vi "Main.vi"(0 "Page Selector":T1, 1 "Code":i32 min=0 max=40000, 5 "Mode Selector":T3, 7 "Instrument Setting":T4={"Error Percentage"=20.0}, 9 "INL Method":T5, 11 "Error In":errorcluster, 12 "Input Voltage Parameters":T6={"Voltage Max"=5.0, "Voltage Min"=0.0, "Resolution (Bits)"=3}) -> (3 "DNL Value":dbl, 4 "Tab Control":T2(tab), 6 "DNL Graph":dbl[](graph), 8 "INL Graph":dbl[](graph), 10 "Ideal Transfer Function":cluster{"Analog Voltage":dbl[], dbl[]}(graph), 13 "INL Value":dbl, 14 "Status":string, 15 "Error Out":errorcluster)   [LabVIEW 2023]
uses:
  Typedef/INL Method.ctl
  Typedef/Page Selector.ctl
  Typedef/Mode Selector.ctl
  Typedef/Input Values.ctl
  Typedef/Instrument Setting.ctl
  Typedef/Queue Operation.ctl
  Typedef/INL DNL Data.ctl
  Classes/Application/Application.lvclass
  Typedef/DVR ref.ctl
  Typedef/User Event Operations.ctl
panel:
  in  "Input":bool
  # "INL AND DNL TESTING INSTRUMENT"
  # "Purpose\nThis tool measures Integral Non-Linearity (INL) and Differential Non-Linearity (DNL) of ADCs and DACs, ensuring accurate linearity performance for various applications.\n\nINL and DNL Definitions\nINL (Integral Non-Linearity): Deviation of the converter's actual transfer function from an ideal straight line.\nDNL (Differential Non-Linearity): Deviation between adjacent digital output levels, indicating the uniformity of steps.\n\nHow to Use\nMode Selection: Choose DAC or ADC.\nInput Parameters: Enter voltage range and bit resolution.\nConfigure Settings: Set error percentage and INL measurement method.\nRun Measurements: View DNL and INL results in real-time."
  # "Please select the mode of the device"
  # "Choose the type of INL Measurement"
  # "Please enter the input voltage parameters to generate ideal transfer function"
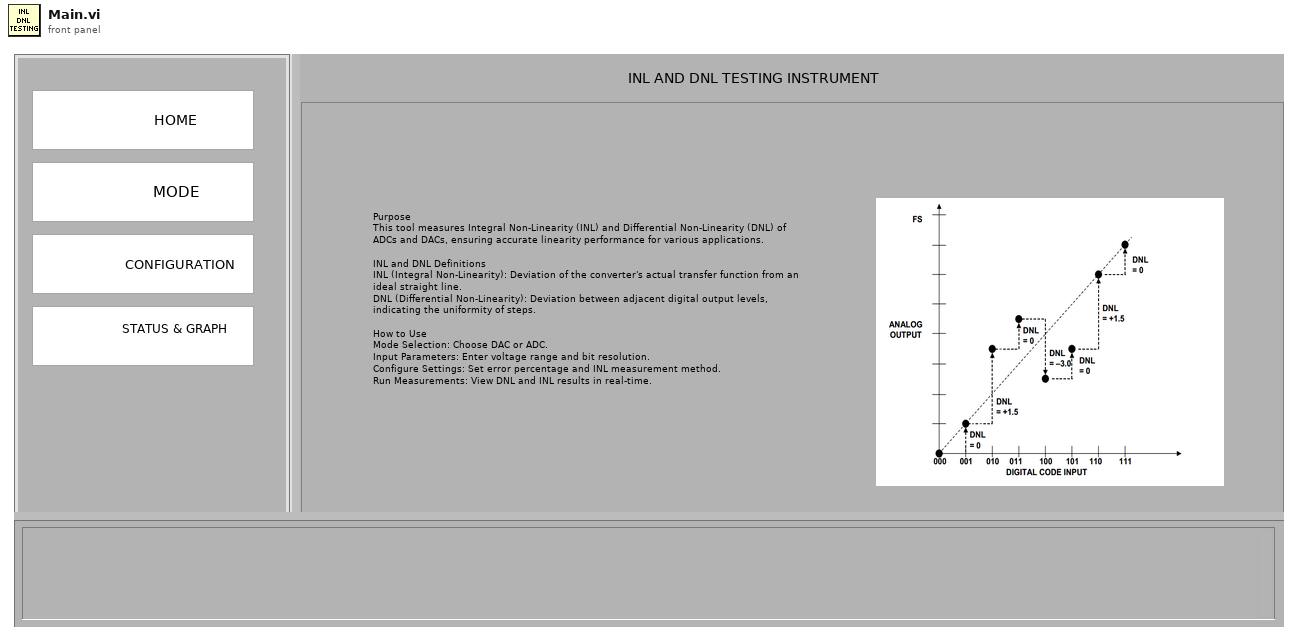
[diagram p1: front panel]
types:
  T1 = typedef "Page Selector.ctl" = cluster{"Mode":bool, "Configuration":bool, "Result":bool, "Home":bool}
  T2 = enum32{"Home Page", "Mode Page", "Configuration Page", "Input Page", "Result Page"}
  T3 = typedef "Mode Selector.ctl" = cluster{"DAC":bool, "ADC":bool}
  T4 = typedef "Instrument Setting.ctl" = cluster{"Error Percentage":dbl}
  T5 = typedef "INL Method.ctl" = enum16{"Best Fit", "End Point"}
  T6 = typedef "Input Values.ctl" = cluster{"Voltage Max":dbl, "Voltage Min":dbl, "Resolution (Bits)":i32}
  T7 = typedef "User Event Operations.ctl" = enum16{"Obtain", "Generate", "Destroy"}
  T8 = typedef "INL DNL Data.ctl" = cluster{"Page":enum32{"Home Page", "Mode Page", "Configuration Page", "Input Page", "Result Page"}, "Voltage Range":dbl, "Input Values":T6, "LSB":dbl, "Analog Voltage":dbl[], "Digital Code":dbl[], "TF Graph":cluster{"Analog Voltage":dbl[], dbl[]}, "DNL":dbl, "INL":dbl, "DNL Graph":dbl[], "Code":i32, "Actual Voltage":dbl[], "INL Graph":dbl[], "V Zero":dbl, "Error Percentage":dbl, "Status Array":string[], "Status Limit":i32, "Statusbar":string, "Active Class":refnum<class "Application.lvclass">, "INL Method":T5, "List of Classes":T9[], "Selected Mode":string, "Base Class":refnum<class "Application.lvclass">}
  T9 = typedef "DVR ref.ctl" = cluster{"Class Name":string, "Class Data":refnum<class "Application.lvclass">}
  T10 = typedef "Queue Operation.ctl" = enum16{"Create & Enqueue N", "Enqueue N", "Dequeue", "Enstack N", "Flush", "Release"}
  T11 = typedef "Queue Element.ctl" = cluster{"State":string, "Data":variant}
  T12 = typedef "Transfer Function.ctl" = cluster{"Ideal voltage":dbl[], "Digital Code":dbl[]}
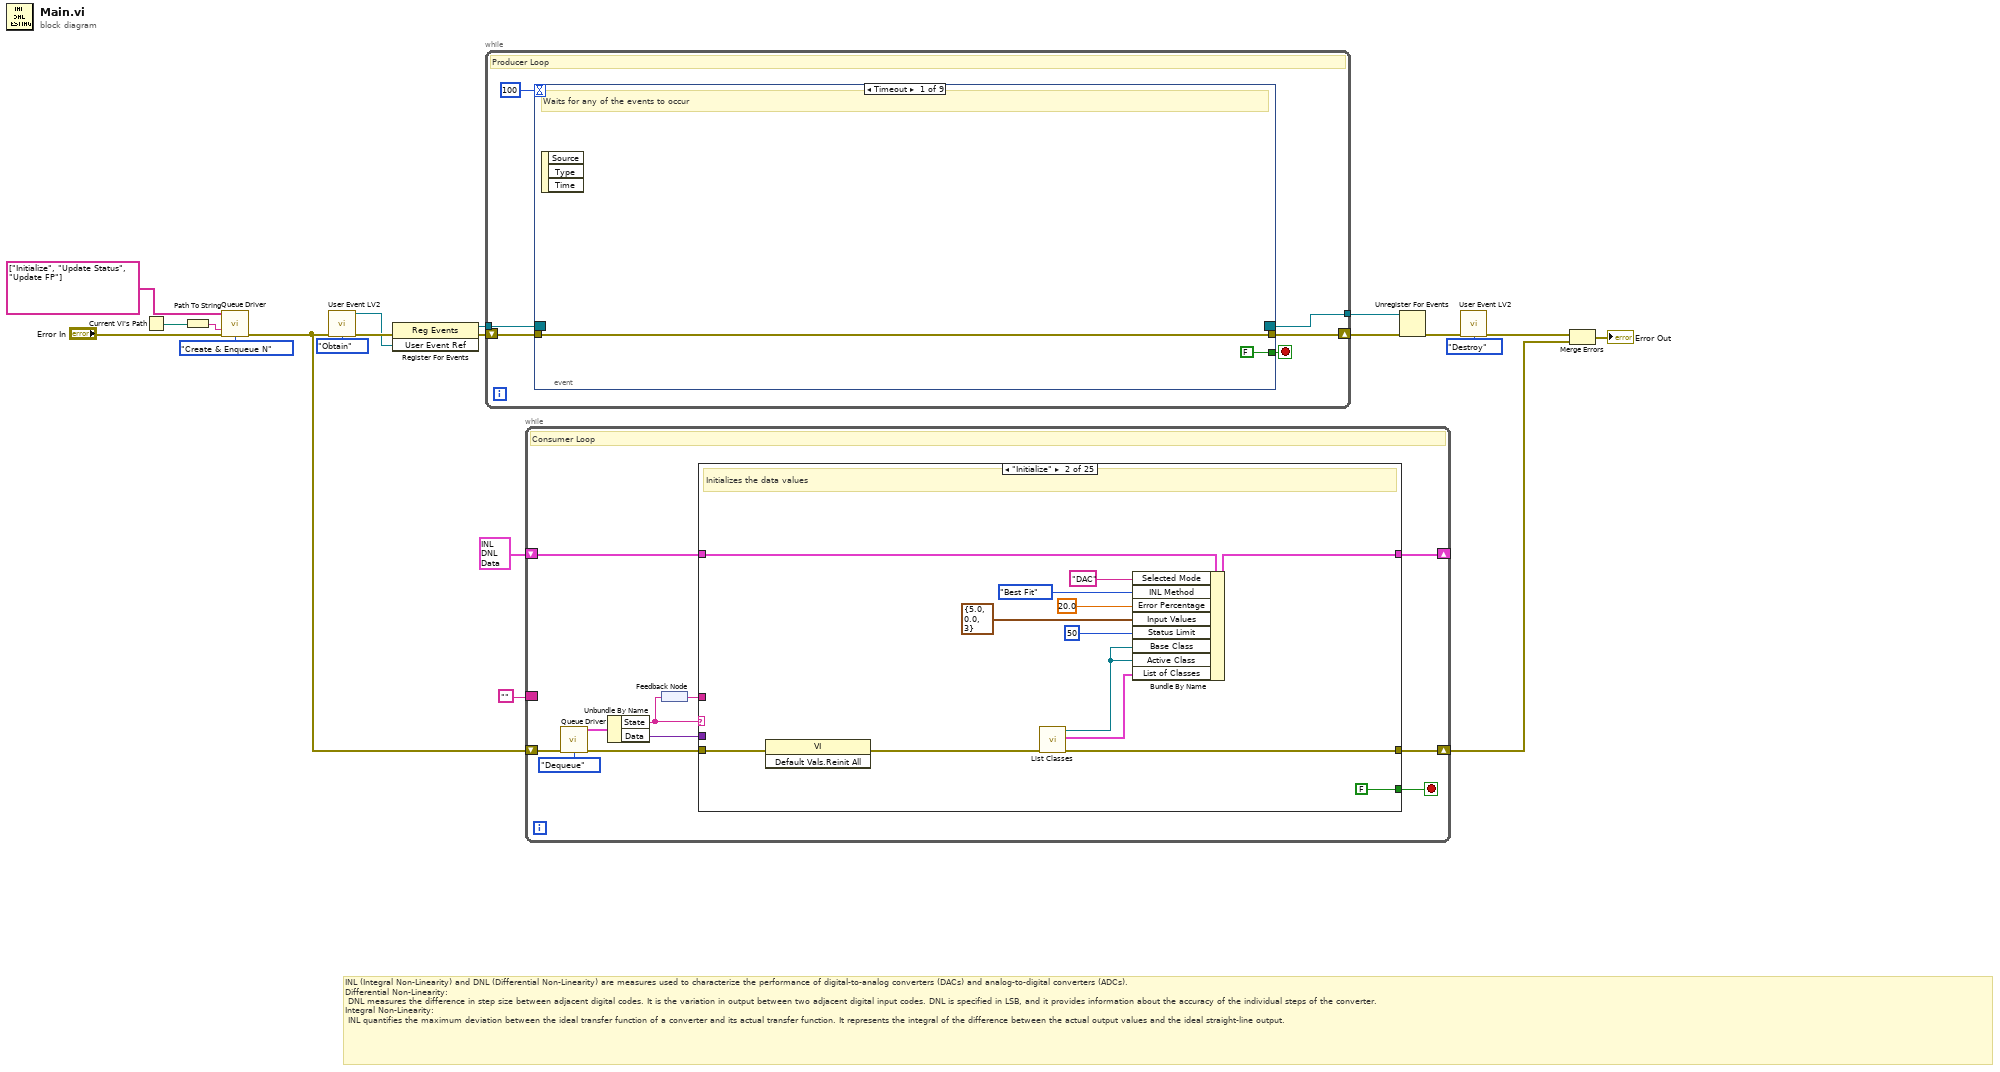
[diagram p0: block diagram]
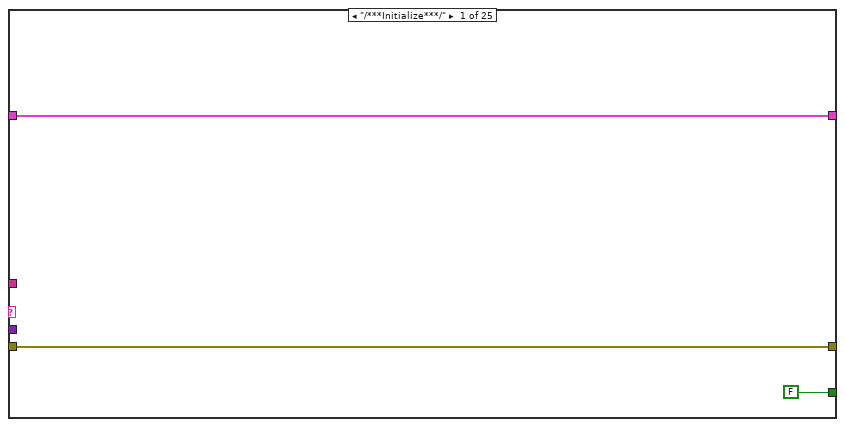
[diagram p2: hidden frame]
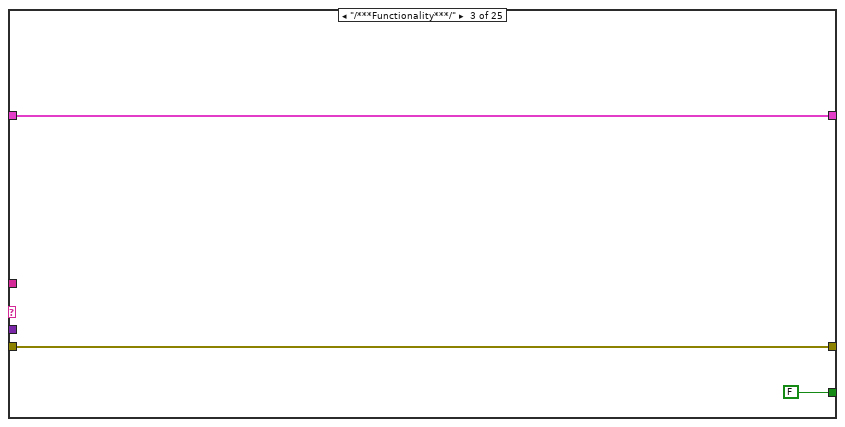
[diagram p3: hidden frame]
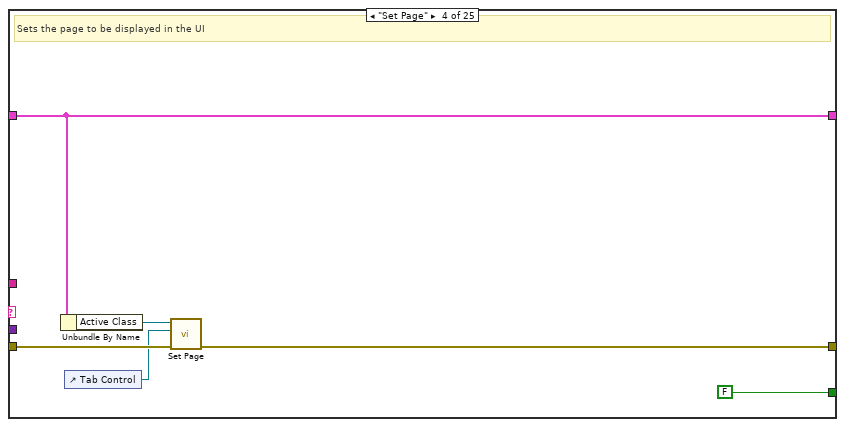
[diagram p4: hidden frame]
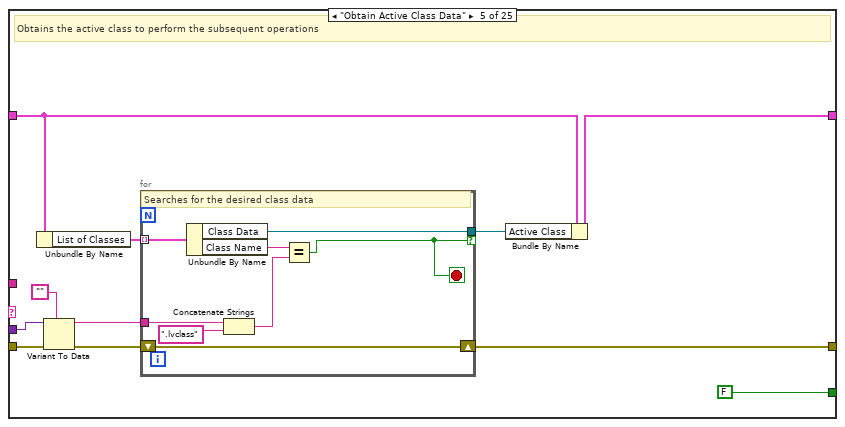
[diagram p5: hidden frame]
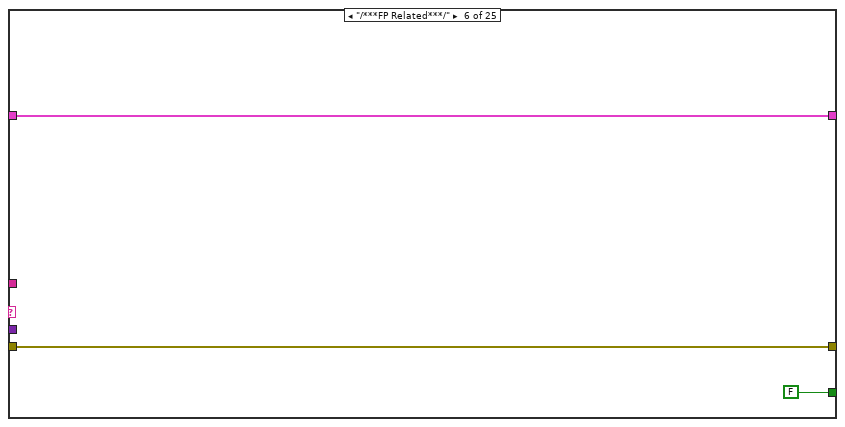
[diagram p6: hidden frame]
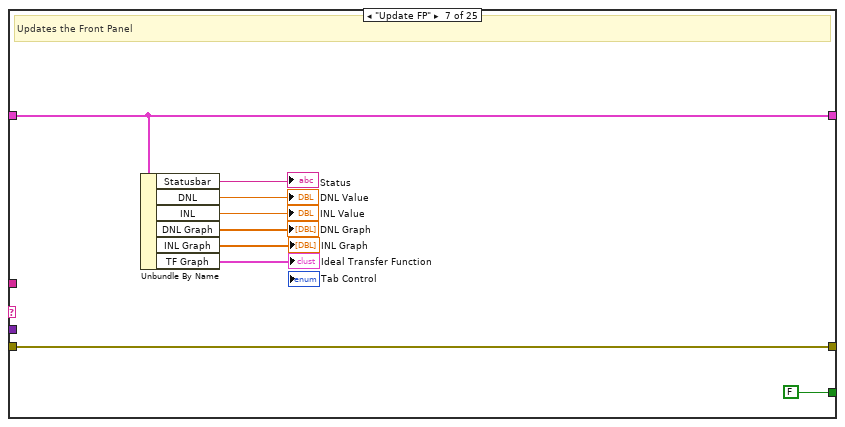
[diagram p7: hidden frame]
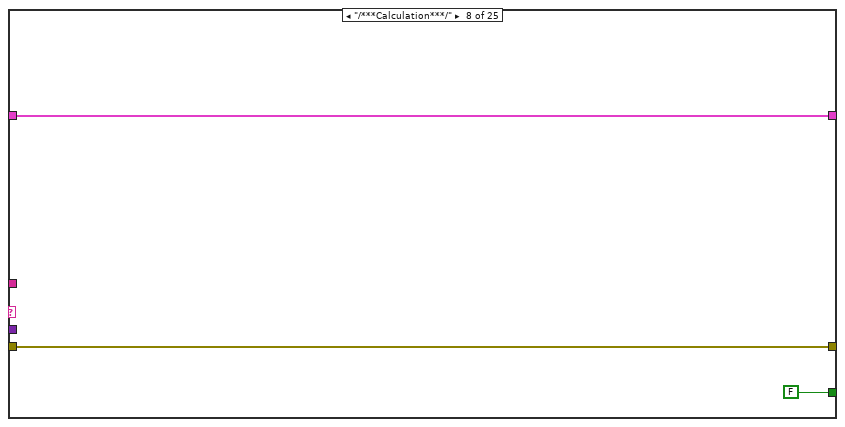
[diagram p8: hidden frame]
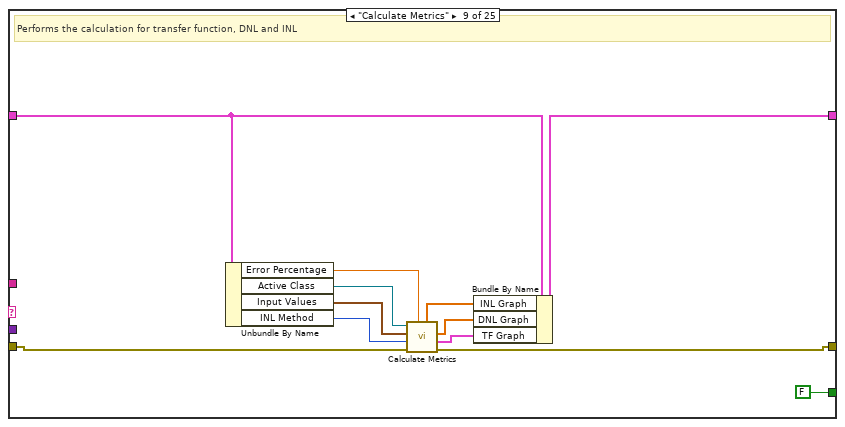
[diagram p9: hidden frame]
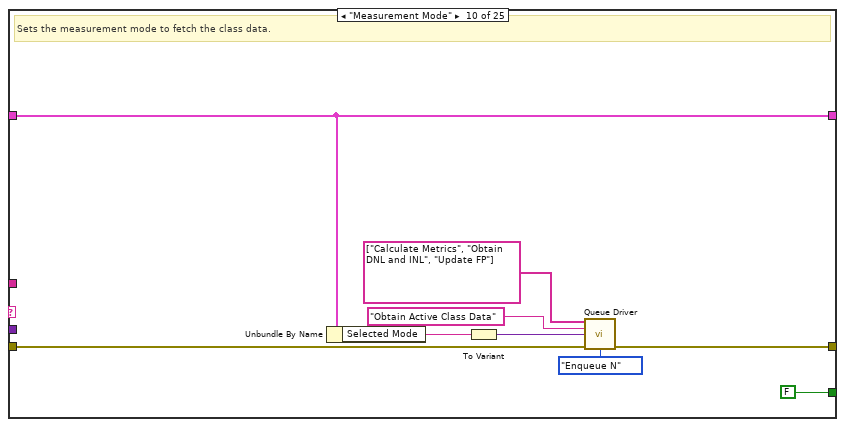
[diagram p10: hidden frame]
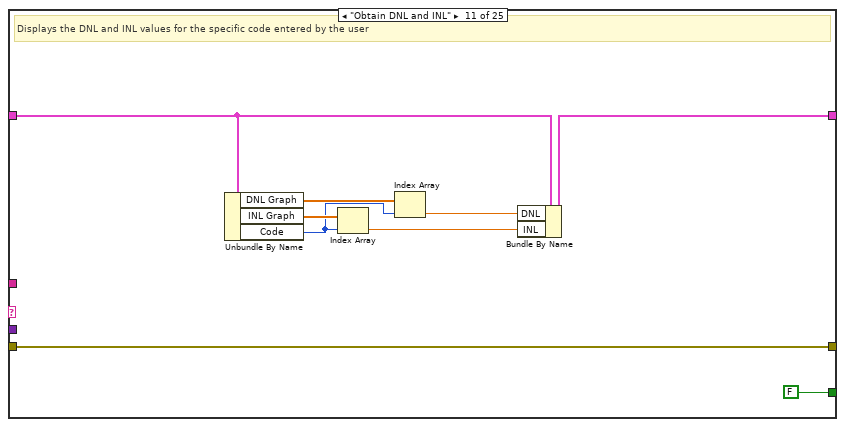
[diagram p11: hidden frame]
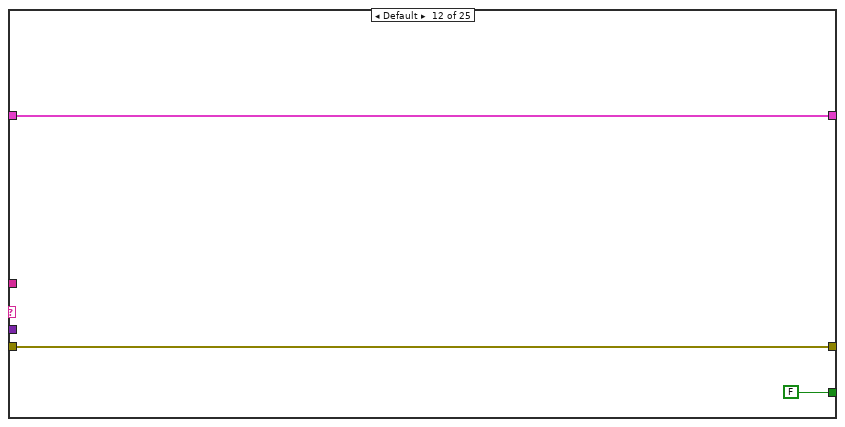
[diagram p12: hidden frame]
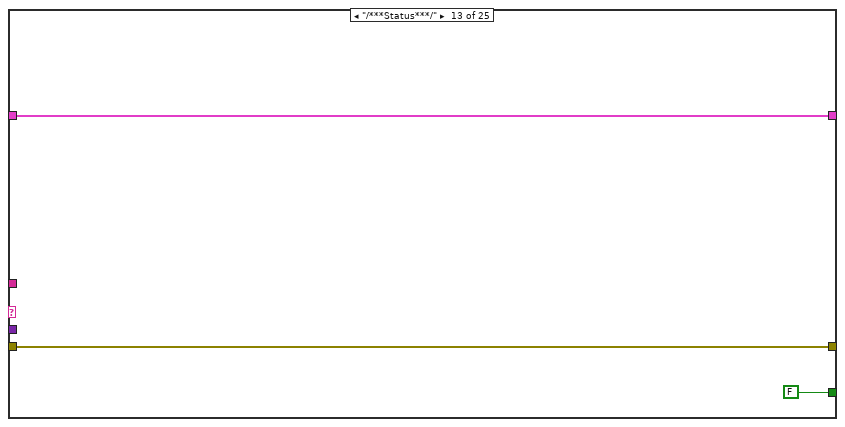
[diagram p13: hidden frame]
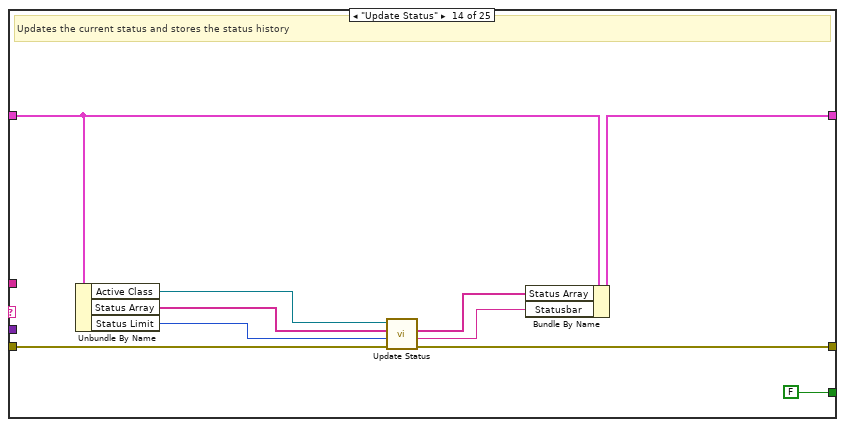
[diagram p14: hidden frame]
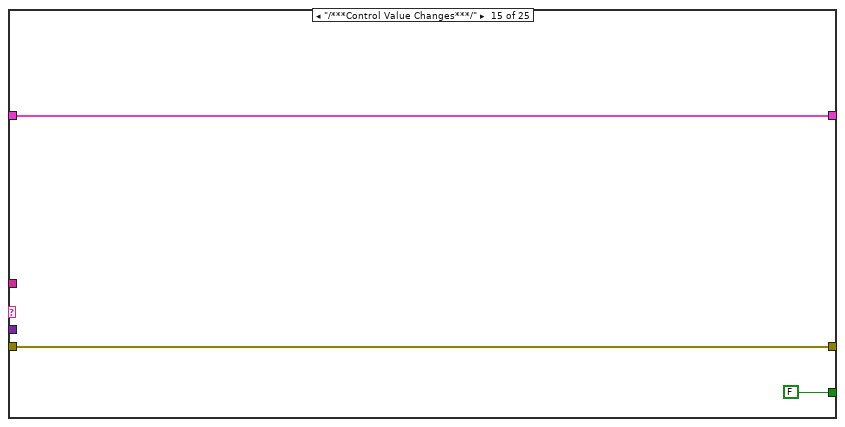
[diagram p15: hidden frame]
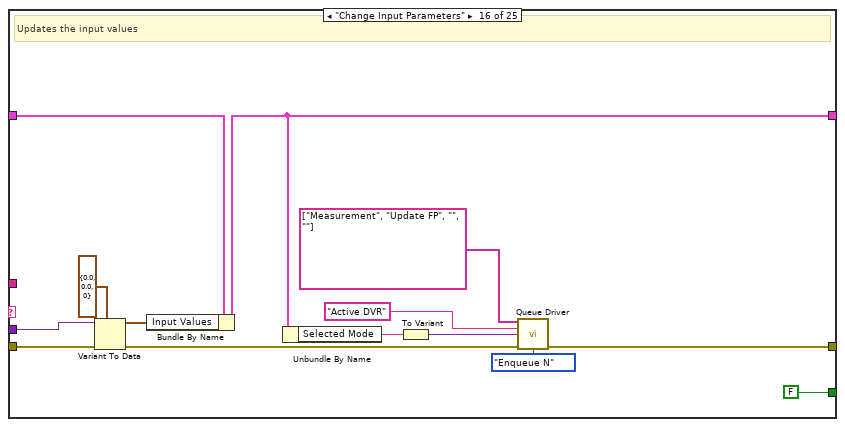
[diagram p16: hidden frame]
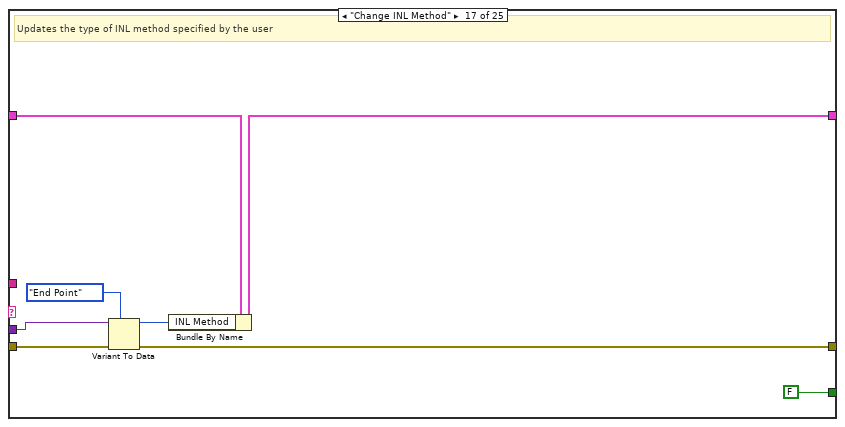
[diagram p17: hidden frame]
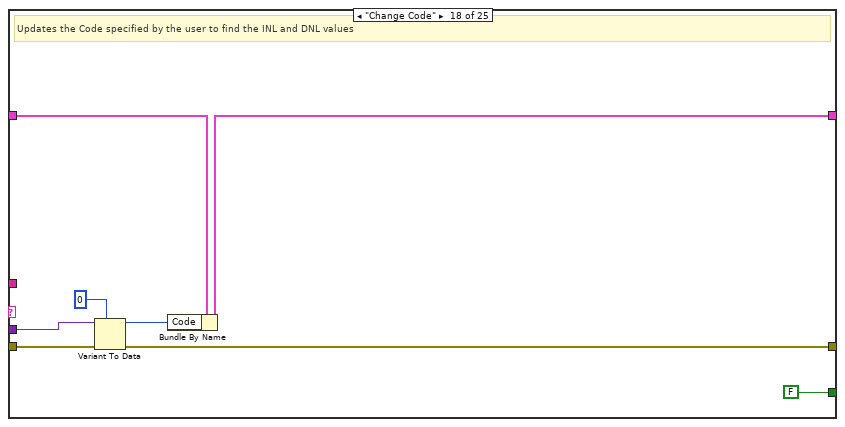
[diagram p18: hidden frame]
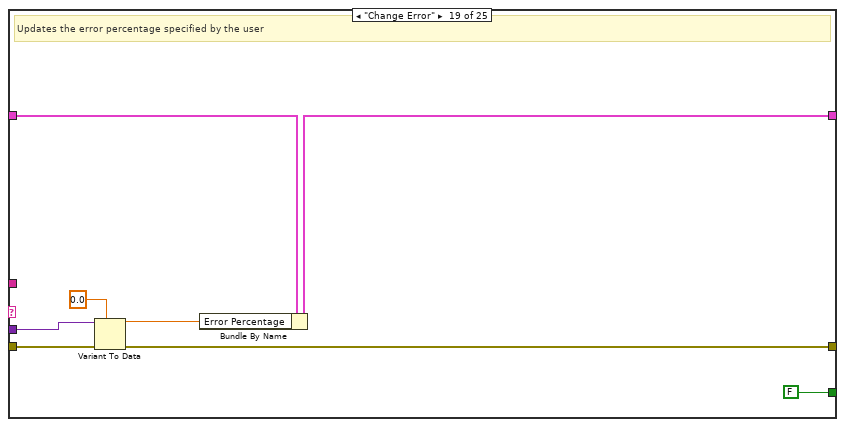
[diagram p19: hidden frame]
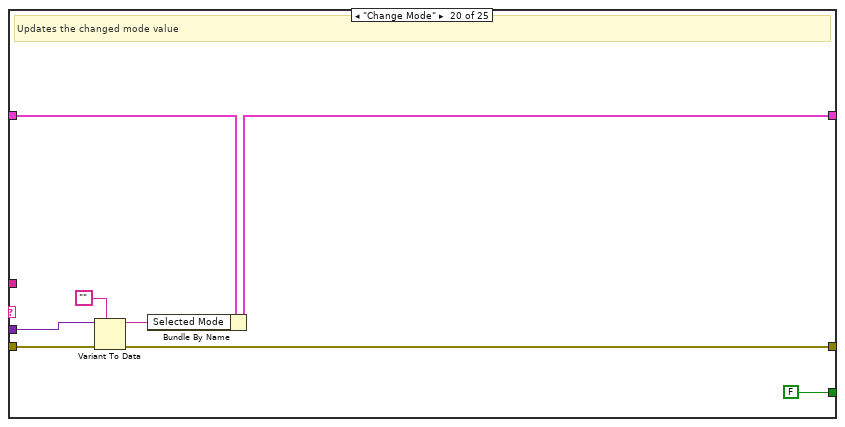
[diagram p20: hidden frame]
diagram:
  # "INL (Integral Non-Linearity) and DNL (Differential Non-Linearity) are measures used to characterize the performance of digital-to-analog converters (DACs) and analog-to-digital converters (ADCs).\nDifferential Non-Linearity:\n DNL measures the difference in step size between adjacent digital codes. It is the variation in output between two adjacent digital input codes. DNL is specified in LSB, and it provides information about the accuracy of the individual steps of the converter.\nIntegral Non-Linearity:\n INL quantifies the maximum deviation between the ideal transfer function of a converter and its actual transfer function. It represents the integral of the difference between the actual output values and the ideal straight-line output."
  n1 = Current VI's Path() -> (path=w5:path)
  n2 = Path To String(path=w5) -> (string=w4:string)
  n3 = call "Queue Driver.vi"("States[]"=string[] ["Initialize", "Update Status", "Update FP"], "Queue Name"=w4, "Error In"="Error In", "Queue Operation"=Queue_Operation."Create & Enqueue N") -> ("Error Out"=w8:errorcluster)  [unwired: 10 in, 1 out]
  n4 = call "User Event LV2.vi"("Error In"=w8, "Operation"=User_Event_Operations."Obtain") -> ("User Event Ref"=w9:refnum<user-event>, "Error Out"=w16:errorcluster)  [unwired: 12 in]
  n5 = register-events(error in=w16, w9) -> (reference out=w14:refnum<event-registration>, error out=w15:errorcluster)  [unwired: 1 in]
  n6 = while {
    shift-right: [w21] -> w20
    shift-left: w15 -> [w26]
    tunnel: w14 -> [w23]
    tunnel: [w22] -> w12
    stop <- w25 stop-if-true
    # "Producer Loop"
    n7 = event shown="[0] Timeout" {
      selector: w23 -> [_ _ _ _ _ _ _ _ _]
      dyn-events: [_ _ _ _ _ _ _ _ _] -> w22
      timeout: 100 -> [_ _ _ _ _ _ _ _ _]
      tunnel: w26 -> [w28 w38 w43 w52 w61 w74 w76 w87 w91]
      tunnel: [FALSE ("Discard?") FALSE ("Stop") FALSE ("Stop") FALSE ("Stop") FALSE ("Stop") FALSE ("Stop") FALSE ("Stop") w83 w89] -> w25
      tunnel: [w28 w30 w42 w51 w57 w71 _ w86 w90] -> w21
      tunnel: [_ _ _ _ _ _ w80 _ _] -> _
      event Timeout {
        # "Waits for any of the events to occur"
        n8 = event-data() -> ()  [unwired: 1 in, 3 out]
      }
      event "Input": Value Change {
        # "Obtains the name of the control clicked and navigates to the respective page"
        n9 = event-data() -> ("CtlRef"=w33:refnum<vi>)  [unwired: 1 in]
        n10 = property class="Bool"(reference=w33, error in=w38) -> (error out=w34:errorcluster, "Label.Text"=w32:string)  [unwired: 1 out]
        n11 = To Variant(anything=w32) -> (Variant=w35:variant)
        n12 = call "Queue Driver.vi"("States[]"=string[] ["Set Page", "Update Status", "Update FP"], "State"="Obtain Active Class Data", "Data"=w35, "Error In"=w34, "Queue Operation"=Queue_Operation."Enqueue N") -> ("Error Out"=w30:errorcluster)  [unwired: 9 in, 1 out]
      }
      event Value Change {
        # "Updates the input voltage paramaters values"
        n13 = event-data() -> ("NewVal"=w45:T6)  [unwired: 1 in]
        n14 = To Variant(anything=w45) -> (Variant=w40:variant)
        n15 = call "Queue Driver.vi"("States[]"=string[] ["Change Input Parameters"], "State"="Input Values", "Data"=w40, "Error In"=w43, "Queue Operation"=Queue_Operation."Enqueue N") -> ("Error Out"=w42:errorcluster)  [unwired: 9 in, 1 out]
      }
      event Value Change {
        # "Updates the type of INL measurement method selected by the user"
        n16 = event-data() -> ("NewVal"=w48:T5)  [unwired: 1 in]
        n17 = To Variant(anything=w48) -> (Variant=w49:variant)
        n18 = call "Queue Driver.vi"("States[]"=string[] ["Measurement Mode"], "State"="Change INL Method", "Data"=w49, "Error In"=w52, "Queue Operation"=Queue_Operation."Enqueue N") -> ("Error Out"=w51:errorcluster)  [unwired: 9 in, 1 out]
      }
      event Value Change {
        # "Obtains the mode selected by the user and triggers to navigate  to the input page."
        n19 = event-data() -> ("CtlRef"=w59:refnum<vi>)  [unwired: 1 in]
        n20 = property class="Bool"(reference=w59, error in=w61) -> (error out=w60:errorcluster, "Label.Text"=w58:string)  [unwired: 1 out]
        n21 = To Variant(anything=w58) -> (Variant=w62:variant)
        n22 = call "Queue Driver.vi"("States[]"=string[] ["Measurement Mode"], "State"="Change Mode", "Data"=w62, "Error In"=w60, "Queue Operation"=Queue_Operation."Enqueue N") -> ("Error Out"=w64:errorcluster)  [unwired: 9 in, 1 out]
        n23 = property on="Input" class="Bool (strict)"(error in=w64, "Val(Sgnl)"=TRUE) -> (error out=w57:errorcluster)  [unwired: 1 in, 1 out]
      }
      event "Code": Value Change {
        # "Updates the new code value to display the INL and DNL values respectively"
        n24 = event-data() -> ("NewVal"=w68:i32)  [unwired: 1 in]
        n25 = To Variant(anything=w68) -> (Variant=w69:variant)
        n26 = call "Queue Driver.vi"("States[]"=string[] ["Obtain DNL and INL", "Update FP"], "State"="Change Code", "Data"=w69, "Error In"=w74, "Queue Operation"=Queue_Operation."Enqueue N") -> ("Error Out"=w71:errorcluster)  [unwired: 9 in, 1 out]
      }
      event Value Change {
        # "Updates the change in error value"
        n27 = event-data() -> ("NewVal"=w77:dbl)  [unwired: 1 in]
        n28 = To Variant(anything=w77) -> (Variant=w78:variant)
        n29 = call "Queue Driver.vi"("States[]"=string[] ["Measurement Mode"], "State"="Change Error", "Data"=w78, "Error In"=w76, "Queue Operation"=Queue_Operation."Enqueue N") -> ("Error Out"=w80:errorcluster)  [unwired: 9 in, 1 out]
      }
      event Panel Close? {
        w84 = TRUE ("Discard?")
        # "Stops the VI running when user clicks panel close"
        n30 = event-data() -> ()  [unwired: 1 in, 1 out]
        n31 = call "Queue Driver.vi"("States[]"=string[] ["Exit"], "Error In"=w87, "Queue Operation"=Queue_Operation."Enstack N") -> ("Error Out"=w86:errorcluster)  [unwired: 11 in, 1 out]
        n32 = event-data("Discard?"=w84) -> ()  [unwired: 1 in, 1 out]
        n33 = Not(x=w84) -> (.not. x?=w83:bool)
      }
      event User Event {
        # "Performs the operation based on the user event"
        n34 = event-data() -> ("Name"=w92:string)  [unwired: 1 in]
        n35 = case shown="\"Stop\"" w92 {
          tunnel: w91 -> [w94 w96]
          tunnel: [w94 w96] -> w90
          tunnel: [FALSE TRUE] -> w89
          frame Default {
          }
          frame "Stop" {
            # "Stops the producer loop"
          }
        }
      }
    }
  }
  n36 = while {
    shift-right: [w107] -> w19
    shift-left: w8 -> [w104]
    border: "" ("State") -> [_]
    shift-right: [w97] -> _
    shift-left: T8 {"Page"=enum."Home Page", "Voltage Range"=0.0, "Input Values"={"Voltage Max"=0.0, "Voltage Min"=0.0, "Resolution (Bits)"=0}, "LSB"=0.0, "Analog Voltage"=[], "Digital Code"=[], "TF Graph"={"Analog Voltage"=[], []}, "DNL"=0.0, "INL"=0.0, "DNL Graph"=[], "Code"=0, "Actual Voltage"=[], "INL Graph"=[], "V Zero"=0.0, "Error Percentage"=0.0, "Status Array"=[], "Status Limit"=0, "Statusbar"="", "Active Class"=refnum, "INL Method"=enum."End Point", "List of Classes"=[], "Selected Mode"="", "Base Class"=refnum} -> [w98]
    stop <- w106 stop-if-true
    # "Consumer Loop"
    n37 = call "Queue Driver.vi"("Error In"=w104, "Queue Operation"=Queue_Operation."Dequeue") -> ("Dequeue Element"=w102:T11, "Error Out"=w103:errorcluster)  [unwired: 12 in]
    n38 = Unbundle By Name(w102) -> ("State"=w100:string, "Data"=w101:variant)
    n39 = feedback-in #1(w100) -> ()
    n40 = feedback #1() -> (w99:string)
    n41 = case shown="\"Initialize\"" w100 {
      tunnel: [w110 w114 w126 w130 w138 w154 w163 w166 w174 w181 w196 w198 w202 w203 w215 w217 w231 w242 w246 w255 w264 w270 w286 w289 w299] -> w107
      tunnel: [FALSE FALSE FALSE FALSE FALSE FALSE FALSE FALSE FALSE FALSE FALSE FALSE FALSE FALSE FALSE FALSE FALSE FALSE FALSE FALSE FALSE FALSE FALSE TRUE FALSE] -> w106
      tunnel: w103 -> [w110 w121 w126 w131 w143 w154 w163 w166 w178 w182 w196 w198 w202 w204 w215 w228 w236 w244 w252 w260 w264 w268 w286 w293 w299]
      tunnel: w101 -> [_ _ _ _ w142 _ _ _ _ _ _ _ _ _ _ w225 w234 w241 w250 w258 _ _ _ _ _]
      tunnel: w99 -> [_ _ _ _ _ _ _ _ _ _ _ _ _ _ _ _ _ _ _ _ _ w269 _ _ _]
      tunnel: w98 -> [w109 w122 w125 w129 w136 w153 w161 w165 w177 w179 w193 w199 w201 w211 w214 w229 w237 w245 w253 w261 w263 w265 w285 w290 w298]
      tunnel: [w109 w120 w125 w129 w134 w153 w161 w165 w175 w179 w194 w199 w201 w210 w214 w220 w230 w240 w247 w257 w263 w265 w285 w290 w298] -> w97
      frame "/***Initialize***/" {
      }
      frame "Initialize" {
        # "Initializes the data values"
        n42 = invoke class="VI" method="Default Vals.Reinit All"(error in=w121) -> (error out=w119:errorcluster)  [unwired: 2 in, 2 out]
        n43 = call "List Classes.vi"("Error In"=w119) -> ("Error Out"=w114:errorcluster, "List of classes"=w113:T9[], "Application Out"=w112:refnum<class "Application.lvclass">)  [unwired: 8 in]
        n44 = Bundle By Name(cluster=w122, "Selected Mode"="DAC", "INL Method"=INL_Method."Best Fit", "Error Percentage"=20.0, "Input Values"=T6 {"Voltage Max"=5.0, "Voltage Min"=0.0, "Resolution (Bits)"=3}, "Status Limit"=50, "Base Class"=w112, "Active Class"=w112, "List of Classes"=w113) -> (w120:T8)
      }
      frame "/***Functionality***/" {
      }
      frame "Set Page" {
        # "Sets the page to be displayed in the UI"
        n45 = Unbundle By Name(w129) -> ("Active Class"=w127:refnum<class "Application.lvclass">)
        n46 = control-ref of="Tab Control"() -> (w128:refnum<vi>)
        n47 = call "Set Page.vi"("Error In"=w131, "Tab Control"=w128, "Application In"=w127) -> ("Error Out"=w130:errorcluster)  [unwired: 7 in, 1 out]
      }
      frame "Obtain Active Class Data" {
        # "Obtains the active class to perform the subsequent operations"
        n48 = Unbundle By Name(w136) -> ("List of Classes"=w135:T9[])
        n49 = Variant To Data(error in=w143, type="", Variant=w142) -> (data=w137:string, error out=w139:errorcluster)
        n50 = for {
          shift-right: [w151] -> w138
          shift-left: w139 -> [w151]
          tunnel: w137 -> [w148]
          tunnel: w135 -> [w150] mode=indexing
          tunnel: [w147] -> w133 if=w146
          stop <- w146 stop-if-true
          # "Searches for the desired class data"
          n51 = Unbundle By Name(w150) -> ("Class Data"=w147:refnum<class "Application.lvclass">, "Class Name"=w149:string)
          n52 = Concatenate Strings(w148, ".lvclass" ("string")) -> (w145:string)
          n53 = Equal?(x=w149, y=w145) -> (x = y?=w146:bool)
        }
        n54 = Bundle By Name(cluster=w136, "Active Class"=w133) -> (w134:T8)
      }
      frame "/***FP Related***/" {
      }
      frame "Update FP" {
        # "Updates the Front Panel"
        n55 = Unbundle By Name(w161) -> ("Statusbar"=→"Status":string, "DNL"=→"DNL Value":dbl, "INL"=→"INL Value":dbl, "DNL Graph"=→"DNL Graph":dbl[], "INL Graph"=→"INL Graph":dbl[], "TF Graph"=→"Ideal Transfer Function":cluster{"Analog Voltage":dbl[], dbl[]})
      }
      frame "/***Calculation***/" {
      }
      frame "Calculate Metrics" {
        # "Performs the calculation for transfer function, DNL and INL"
        n56 = Unbundle By Name(w177) -> ("Error Percentage"=w167:dbl, "Active Class"=w173:refnum<class "Application.lvclass">, "Input Values"=w172:T6, "INL Method"=w168:T5)
        n57 = call "Calculate Metrics.vi"("Error Percentage"=w167, "Error In"=w178, "INL Method"=w168, "Input Values"=w172, "Application In"=w173) -> ("Error Out"=w174:errorcluster, "Transfer Function"=w171:T12, "DNL Values"=w170:dbl[], "INL Values"=w169:dbl[])  [unwired: 2 in, 1 out]
        n58 = Bundle By Name(cluster=w177, "INL Graph"=w169, "DNL Graph"=w170, "TF Graph"=w171) -> (w175:T8)
      }
      frame "Measurement Mode" {
        # "Sets the measurement mode to fetch the class data."
        n59 = Unbundle By Name(w179) -> ("Selected Mode"=w183:string)
        n60 = To Variant(anything=w183) -> (Variant=w186:variant)
        n61 = call "Queue Driver.vi"("States[]"=string[] ["Calculate Metrics", "Obtain DNL and INL", "Update FP"], "State"="Obtain Active Class Data", "Data"=w186, "Error In"=w182, "Queue Operation"=Queue_Operation."Enqueue N") -> ("Error Out"=w181:errorcluster)  [unwired: 9 in, 1 out]
      }
      frame "Obtain DNL and INL" {
        # "Displays the DNL and INL values for the specific code entered by the user"
        n62 = Unbundle By Name(w193) -> ("DNL Graph"=w191:dbl[], "INL Graph"=w192:dbl[], "Code"=w190:i32)
        n63 = Index Array(array=w192, index=w190) -> (element=w188:dbl)
        n64 = Index Array(array=w191, index=w190) -> (element=w189:dbl)
        n65 = Bundle By Name(cluster=w193, "DNL"=w189, "INL"=w188) -> (w194:T8)
      }
      frame Default {
      }
      frame "/***Status***/" {
      }
      frame "Update Status" {
        # "Updates the current status and stores the status history"
        n66 = Unbundle By Name(w211) -> ("Active Class"=w207:refnum<class "Application.lvclass">, "Status Array"=w208:string[], "Status Limit"=w209:i32)
        n67 = call "Update Status.vi"("Error In"=w204, "Status Limit"=w209, "Status History In"=w208, "Application In"=w207) -> ("Error Out"=w203:errorcluster, "Status"=w205:string, "Status History Out"=w206:string[])  [unwired: 2 in, 1 out]
        n68 = Bundle By Name(cluster=w211, "Status Array"=w206, "Statusbar"=w205) -> (w210:T8)
      }
      frame "/***Control Value Changes***/" {
      }
      frame "Change Input Parameters" {
        # "Updates the input values"
        n69 = Variant To Data(error in=w228, type=T6 {"Voltage Max"=0.0, "Voltage Min"=0.0, "Resolution (Bits)"=0} ("Input Values"), Variant=w225) -> (data=w223:T6, error out=w226:errorcluster)
        n70 = Bundle By Name(cluster=w229, "Input Values"=w223) -> (w220:T8)
        n71 = Unbundle By Name(w220) -> ("Selected Mode"=w219:string)
        n72 = To Variant(anything=w219) -> (Variant=w218:variant)
        n73 = call "Queue Driver.vi"("States[]"=string[] ["Measurement", "Update FP", "", ""], "State"="Active DVR", "Data"=w218, "Error In"=w226, "Queue Operation"=Queue_Operation."Enqueue N") -> ("Error Out"=w217:errorcluster)  [unwired: 9 in, 1 out]
      }
      frame "Change INL Method" {
        # "Updates the type of INL method specified by the user"
        n74 = Variant To Data(error in=w236, type=INL_Method."End Point" ("NewVal"), Variant=w234) -> (data=w232:T5, error out=w231:errorcluster)
        n75 = Bundle By Name(cluster=w237, "INL Method"=w232) -> (w230:T8)
      }
      frame "Change Code" {
        # "Updates the Code specified by the user to find the INL and DNL values"
        n76 = Variant To Data(error in=w244, type=0 ("Code"), Variant=w241) -> (data=w239:i32, error out=w242:errorcluster)
        n77 = Bundle By Name(cluster=w245, "Code"=w239) -> (w240:T8)
      }
      frame "Change Error" {
        # "Updates the error percentage specified by the user"
        n78 = Variant To Data(error in=w252, type=0.0 ("Code"), Variant=w250) -> (data=w249:dbl, error out=w246:errorcluster)
        n79 = Bundle By Name(cluster=w253, "Error Percentage"=w249) -> (w247:T8)
      }
      frame "Change Mode" {
        # "Updates the changed mode value"
        n80 = Variant To Data(error in=w260, type="", Variant=w258) -> (data=w254:string, error out=w255:errorcluster)
        n81 = Bundle By Name(cluster=w261, "Selected Mode"=w254) -> (w257:T8)
      }
      frame "/***Error***/" {
      }
      frame "Error" {
        # "Handles the error based on the user acknowledgement"
        n82 = Unbundle By Name(w268) -> ("code"=w267:i32, "source"=w266:string)
        n83 = call <vilib>:"Clear Errors.vi"("error in (no error)"=w268) -> ("error out"=w277:errorcluster)  [unwired: 5 in, 1 out]
        n84 = Format Into String(format string="Error occurred in state \"%s\"!!\nError Code: %d\nError Source: %s\n\nDo you wish to continue?", error in=w277, w269, w267, w266) -> (resulting string=w275:string, error out=w271:errorcluster)  [unwired: 1 in]
        n85 = Two Button Dialog(message=w275, 1:"Exit" ("F button name (\"Cancel\")"), 2:"Continue" ("T button name (\"OK\")")) -> (T button?=w272:bool)
        n86 = case "Continue?" shown="False" w272 {
          tunnel: w271 -> [w282 w283]
          tunnel: [w281 w283] -> w270
          frame False {
            # "Enqueues exit state to stop the VI running"
            n87 = call "Queue Driver.vi"("States[]"=string[] ["Exit"], "Error In"=w282, "Queue Operation"=Queue_Operation."Enstack N") -> ("Error Out"=w281:errorcluster)  [unwired: 11 in, 1 out]
          }
          frame True {
            # "Continues the process"
          }
        }
      }
      frame "/***Exit***/" {
      }
      frame "Exit" {
        # "Releases the queue and stops the consumer loop running"
        n88 = call "Queue Driver.vi"("Error In"=w293, "Queue Operation"=Queue_Operation."Flush") -> ("Error Out"=w292:errorcluster)  [unwired: 12 in, 1 out]
        n89 = call "Queue Driver.vi"("Error In"=w292, "Queue Operation"=Queue_Operation."Release") -> ("Error Out"=w291:errorcluster)  [unwired: 12 in, 1 out]
        n90 = call "User Event LV2.vi"("Event Name"="Stop", "Error In"=w291, "Operation"=User_Event_Operations."Generate") -> ("Error Out"=w289:errorcluster)  [unwired: 11 in, 1 out]
      }
      frame "" {
      }
    }
  }
  n91 = Unregister For Events(event registration refnum=w12, error in=w20) -> (error out=w13:errorcluster)
  n92 = call "User Event LV2.vi"("Error In"=w13, "Operation"=User_Event_Operations."Destroy") -> ("Error Out"=w11:errorcluster)  [unwired: 12 in, 1 out]
  n93 = Merge Errors(w11, w19) -> (→"Error Out":errorcluster)
